vi "Get User Input_Original.vi"(1 "Serial Number In":string) -> (0 "fXpgIdentity Output":T1)   [LabVIEW 2010]
panel:
  in  "Device FIRMWARE VERSION":u16(ring) items=["R1.00.0004", "R1.00.0005", "--Choose--"]
  in  "Continue Button":bool
  in  "Device MICS ID":u32 format="%06x"
  in  "Device SERIAL Number":string
  in  "Device LOT Number":string
  # "Enter All Device Parameters Below.\nWhen finished, click \"Continue\"."
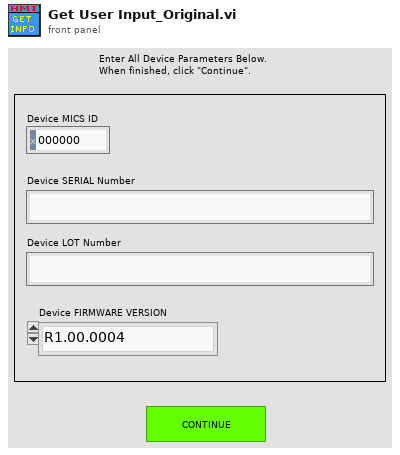
[diagram p1: front panel]
types:
  T1 = cluster{"micsID":u32, "xpgLotNumber":string, "xpgSerialNumber[20]":string, "xpgFirmwareVersion":string}
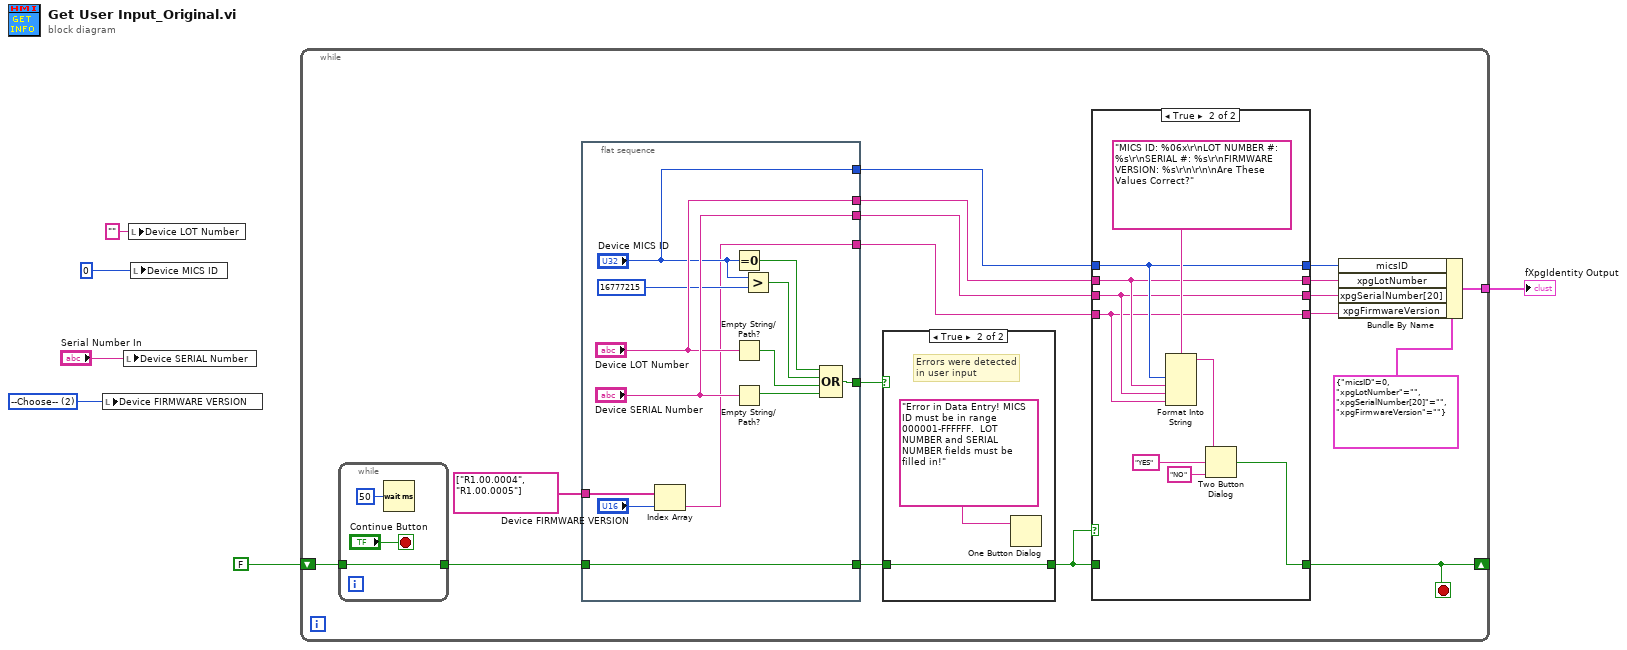
[diagram p0: block diagram]
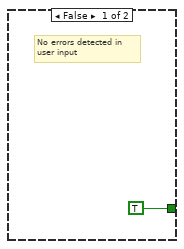
[diagram p3: hidden frame]
diagram:
  w2 = u16 2 items=["R1.00.0004", "R1.00.0005", "--Choose--"] ("Device FIRMWARE VERSION")
  n1 = local write "Device FIRMWARE VERSION"(w2) -> ()
  n2 = local write "Device SERIAL Number"("Serial Number In") -> ()
  n3 = local write "Device LOT Number"("" ("Device LOT Number")) -> ()
  n4 = local write "Device MICS ID"(u32 0 ("Device MICS ID")) -> ()
  n5 = while {
    shift-right: [w16] -> _
    shift-left: FALSE -> [w23]
    tunnel: [w14] -> w1
    stop <- w16 stop-if-true
    n6 = while {
      tunnel: w23 -> [w56]
      tunnel: [w56] -> w21
      stop <- "Continue Button" stop-if-true
      n7 = Wait (ms)(milliseconds to wait=u32 50) -> ()  [unwired: 1 out]
    }
    n8 = flat-sequence {
      tunnel: [w48] -> w22
      tunnel: ["Device SERIAL Number"] -> w17
      tunnel: ["Device LOT Number"] -> w18
      tunnel: ["Device MICS ID"] -> w11
      tunnel: w21 -> [w45]
      tunnel: [w45] -> w20
      tunnel: string[] ["R1.00.0004", "R1.00.0005"] -> [w39]
      tunnel: [w38] -> w8
      frame #0 {
        n9 = Index Array(array=w39, index="Device FIRMWARE VERSION") -> (element=w38:string)
        n10 = Equal To 0?(x="Device MICS ID") -> (x = 0?=w42:bool)
        n11 = Empty String/Path?(string/path="Device LOT Number") -> (empty?=w49:bool)
        n12 = Empty String/Path?(string/path="Device SERIAL Number") -> (empty?=w50:bool)
        n13 = Greater?(x="Device MICS ID", y=u32 16777215) -> (0:w41:bool)
        n14 = Compound Arithmetic op=OR(w42, w41, w49, w50) -> (w48:bool)
      }
    }
    n15 = case shown="True" w22 {
      tunnel: w20 -> [_ w53]
      tunnel: [TRUE w53] -> w19
      frame False {
        # "No errors detected in\nuser input"
      }
      frame True {
        # "Errors were detected\nin user input"
        n16 = One Button Dialog(message="Error in Data Entry! MICS ID must be in range 000001-FFFFFF.  LOT NUMBER and SERIAL NUMBER fields must be filled in!") -> ()  [unwired: 1 in, 1 out]
      }
    }
    n17 = case shown="True" w19 {
      tunnel: w19 -> [w28 _]
      tunnel: w11 -> [w27 w32]
      tunnel: w18 -> [w26 w31]
      tunnel: w17 -> [w25 w30]
      tunnel: [w28 w33] -> w16
      tunnel: [w27 w32] -> w10
      tunnel: [w26 w31] -> w13
      tunnel: [w25 w30] -> w12
      tunnel: w8 -> [w24 w29]
      tunnel: [w24 w29] -> w7
      frame False {
      }
      frame True {
        n18 = Format Into String(format string="MICS ID: %06x\r\nLOT NUMBER #: %s\r\nSERIAL #: %s\r\nFIRMWARE VERSION: %s\r\n\r\n\nAre These Values Correct?", w32, w31, w30, w29) -> (resulting string=w36:string)  [unwired: 2 in, 1 out]
        n19 = Two Button Dialog(message=w36, 1:"NO" ("F button name (\"Cancel\")"), 2:"YES" ("T button name (\"OK\")")) -> (T button?=w33:bool)
      }
    }
    n20 = Bundle By Name(cluster=T1 {"micsID"=0, "xpgLotNumber"="", "xpgSerialNumber[20]"="", "xpgFirmwareVersion"=""} ("fXpgIdentity Output"), "micsID"=w10, "xpgLotNumber"=w13, "xpgSerialNumber[20]"=w12, "xpgFirmwareVersion"=w7) -> (w14:T1)
  }
  "fXpgIdentity Output" <- w1
